vi "DAC Save Results.vi"(8 "error in":errorcluster, 9 "Log Details?":bool, 10 "tdms file":refnum<k34>, 11 "DAC HeatFlow Load dU in":refnum<class "DAC HeatFlow Load dU.lvclass">) -> (0 "error out":errorcluster)   [LabVIEW 2019, in "DAC.lvlib" / "DAC HeatFlow Load dU.lvclass"]
uses:
  DAC HeatFlow Load dU.lvclass
  C:/Users/krio/Documents/LV_Projects/test-stand/App/DAC/DAC.lvclass
  DAC.lvclass/DAC.ctl
  DAC HeatFlow Load dU.lvclass/DAC HeatFlow Load dU.ctl
  DAC.lvclass
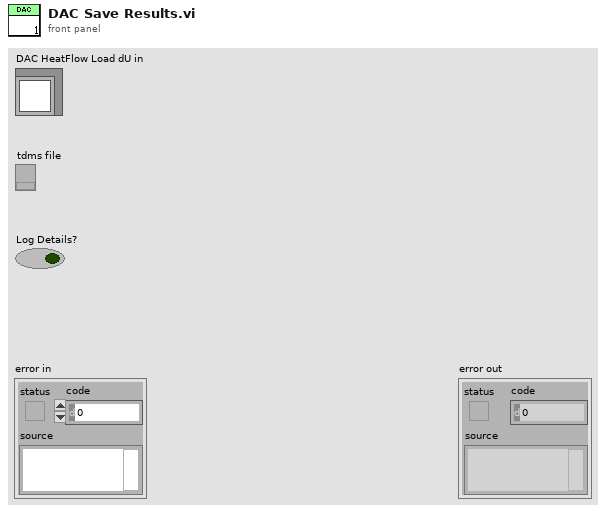
[diagram p1: front panel]
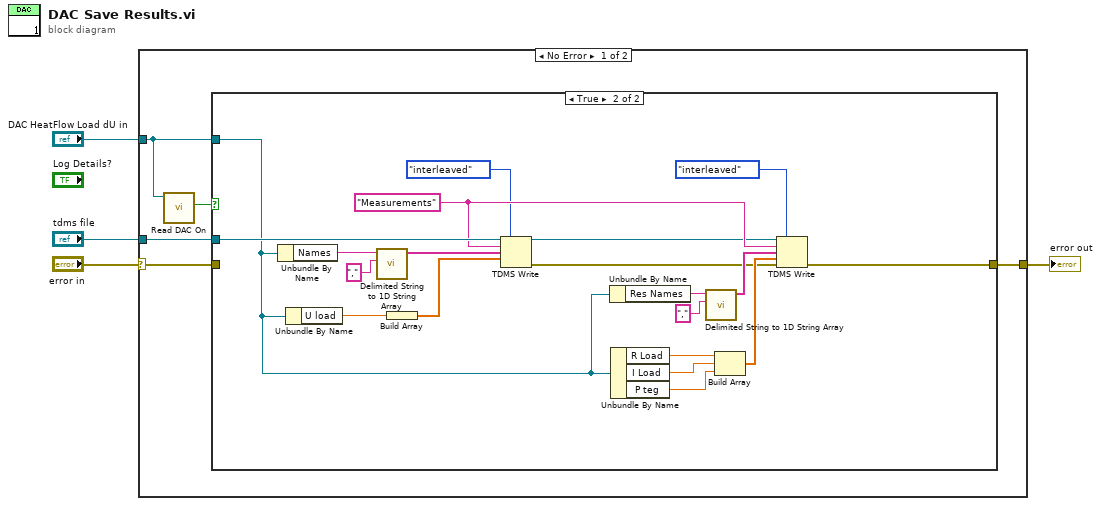
[diagram p0: block diagram]
diagram:
  n1 = case shown="No Error" "error in" {
    selector: "error in" -> [w6 w31]
    tunnel: "DAC HeatFlow Load dU in" -> [w9 _]
    tunnel: "tdms file" -> [w7 _]
    tunnel: [w5 w31] -> w1
    frame No Error {
      n2 = call "Read DAC On.vi"("DAC in"=w9) -> ("DAC On"=w8:bool)  [unwired: 8 in, 2 out]
      n3 = case shown="True" w8 {
        tunnel: w9 -> [_ w14]
        tunnel: w7 -> [_ w30]
        tunnel: w6 -> [w10 _]
        tunnel: [w10 w20] -> w5
        frame False {
        }
        frame True {
          w29 = "Measurements" ("group name in (Untitled)")
          n4 = Unbundle By Name(w14) -> ("Names"=w18:string)
          n5 = Unbundle By Name(w14) -> ("U load"=w17:dbl)
          n6 = call <vilib>:"Delimited String to 1D String Array.vi"("delimiter"=",", "delimited string"=w18) -> ("string array"=w16:string[])  [unwired: 9 in]
          n7 = Build Array(w17) -> (w15:dbl[])
          n8 = TDMS Write(0:w30, 1:enum16{"decimated", "interleaved"}."interleaved" ("data layout (0:decimated)"), 5:w29, 7:w16, 9:w15) -> (4:w13:refnum<k34>, 15:w21:errorcluster)  [unwired: 1 in, 2 out]
          n9 = Unbundle By Name(w14) -> ("Res Names"=w27:string)
          n10 = Unbundle By Name(w14) -> ("R Load"=w25:dbl, "I Load"=w24:dbl, "P teg"=w23:dbl)
          n11 = call <vilib>:"Delimited String to 1D String Array.vi"("delimiter"=",", "delimited string"=w27) -> ("string array"=w26:string[])  [unwired: 9 in]
          n12 = Build Array(w25, w24, w23) -> (w22:dbl[])
          n13 = TDMS Write(0:w13, 1:enum16{"decimated", "interleaved"}."interleaved" ("data layout (0:decimated)"), 5:w29, 7:w26, 9:w22, 11:w21) -> (15:w20:errorcluster)  [unwired: 3 out]
        }
      }
    }
    frame Error {
    }
  }
  "error out" <- w1
